vi "Func-엑셀 데이터를 그래프로 출력.vi"() -> ()   [LabVIEW 2015] (continued)
930.01\n930.03\n930.04\n930.06\n930.08\n930.09\n930.11\n930.13\n930.14\n930.16\n930.18\n930.2\n930.21\n930.23\n930.25\n930.26\n930.28\n930.29\n930.31\n930.33\n930.34\n930.36\n930.38\n930.39\n930.41\n930.43\n930.44\n930.46\n930.48\n930.49\n930.51\n930.53\n930.54\n930.56\n930.58\n930.59\n930.61\n930.63\n930.64\n930.66\n930.68\n930.69\n930.71\n930.73\n930.74\n930.76\n930.78\n930.79\n930.81\n930.83\n930.84\n930.86\n930.88\n930.89\n930.91\n930.93\n930.94\n930.96\n930.98\n930.99\n931.01\n931.03\n931.04\n931.06\n931.08\n931.09\n931.11\n931.13\n931.14\n931.16\n931.18\n931.19\n931.21\n931.23\n931.24\n931.26\n931.28\n931.29\n931.31\n931.33\n931.34\n931.36\n931.38\n931.39\n931.41\n931.43\n931.44\n931.46\n931.48\n931.49\n931.51\n931.53\n931.54\n931.56\n931.58\n931.59\n931.61\n931.63\n931.65\n931.66\n931.68\n931.69\n931.71\n931.73\n931.75\n931.76\n931.78\n931.79\n931.81\n931.83\n931.84\n931.86\n931.88\n931.9\n931.91\n931.93\n931.94\n931.96\n931.98\n932\n932.01\n932.03\n932.04\n932.06\n932.08\n932.1\n932.11\n932.13\n932.14\n932.16\n932.18\n932.19\n932.21\n932.23\n932.25\n932.26\n932.28\n932.29\n932.31\n932.33\n932.35\n932.36\n932.38\n932.39\n932.41\n932.43\n932.44\n932.46\n932.48\n932.49\n932.51\n932.53\n932.54\n932.56\n932.58\n932.59\n932.61\n932.63\n932.64\n932.66\n932.68\n932.69\n932.71\n932.73\n932.74\n932.76\n932.78\n932.79\n932.81\n932.83\n932.84\n932.86\n932.88\n932.89\n932.91\n932.93\n932.94\n932.96\n932.98\n932.99\n933.01\n933.03\n933.04\n933.06\n933.08\n933.09\n933.11\n933.13\n933.14\n933.16\n933.18\n933.19\n933.21\n933.23\n933.24\n933.26\n933.28\n933.29\n933.31\n933.33\n933.34\n933.36\n933.38\n933.39\n933.41\n933.43\n933.44\n933.46\n933.48\n933.49\n933.51\n933.53\n933.54\n933.56\n933.58\n933.59\n933.61\n933.63\n933.64\n933.66\n933.68\n933.69\n933.71\n933.73\n933.74\n933.76\n933.78\n933.79\n933.81\n933.83\n933.84\n933.86\n933.88\n933.89\n933.91\n933.93\n933.94\n933.96\n933.98\n933.99\n934.01\n934.03\n934.04\n934.06\n934.08\n934.09\n934.11\n934.13\n934.14\n934.16\n934.18\n934.19\n934.21\n934.23\n934.24\n934.26\n934.28\n934.29\n934.31\n934.33\n934.34\n934.36\n934.38\n934.4\n934.41\n934.43\n934.44\n934.46\n934.48\n934.49\n934.51\n934.53\n934.54\n934.56\n934.58\n934.59\n934.61\n934.63\n934.65\n934.66\n934.68\n934.69\n934.71\n934.73\n934.75\n934.76\n934.78\n934.79\n934.81\n934.83\n934.84\n934.86\n934.88\n934.89\n934.91\n934.93\n934.94\n934.96\n934.98\n935\n935.01\n935.03\n935.04\n935.06\n935.08\n935.1\n935.11\n935.13\n935.14\n935.16\n935.18\n935.2\n935.21\n935.23\n935.24\n935.26\n935.28\n935.29\n935.31\n935.33\n935.35\n935.36\n935.38\n935.39\n935.41\n935.43\n935.45\n935.46\n935.48\n935.49\n935.51\n935.53\n935.54\n935.56\n935.58\n935.6\n935.61\n935.63\n935.64\n935.66\n935.68\n935.7\n935.71\n935.73\n935.74\n935.76\n935.78\n935.8\n935.81\n935.83\n935.84\n935.86\n935.88\n935.89\n935.91\n935.93\n935.94\n935.96\n935.98\n935.99\n936.01\n936.03\n936.04\n936.06\n936.08\n936.09\n936.11\n936.13\n936.14\n936.16\n936.18\n936.19\n936.21\n936.23\n936.24\n936.26\n936.28\n936.29\n936.31\n936.33\n936.34\n936.36\n936.38\n936.39\n936.41\n936.43\n936.44\n936.46\n936.48\n936.49\n936.51\n936.53\n936.54\n936.56\n936.58\n936.59\n936.61\n936.63\n936.64\n936.66\n936.68\n936.69\n936.71\n936.73\n936.74\n936.76\n936.78\n936.79\n936.81\n936.83\n936.84\n936.86\n936.88\n936.89\n936.91\n936.93\n936.94\n936.96\n936.98\n936.99\n937.01\n937.03\n937.04\n937.06\n937.08\n937.09\n937.11\n937.13\n937.14\n937.16\n937.18\n937.19\n937.21\n937.23\n937.24\n937.26\n937.28\n937.29\n937.31\n937.33\n937.34\n937.36\n937.38\n937.4\n937.41\n937.43\n937.44\n937.46\n937.48\n937.5\n937.51\n937.53\n937.54\n937.56\n937.58\n937.59\n937.61\n937.63\n937.65\n937.66\n937.68\n937.69\n937.71\n937.73\n937.75\n937.76\n937.78\n937.79\n937.81\n937.83\n937.85\n937.86\n937.88\n937.89\n937.91\n937.93\n937.94\n937.96\n937.98\n937.99\n938.01\n938.03\n938.04\n938.06\n938.08\n938.1\n938.11\n938.13\n938.14\n938.16\n938.18\n938.2\n938.21\n938.23\n938.24\n938.26\n938.28\n938.29\n938.31\n938.33\n938.35\n938.36\n938.38\n938.39\n938.41\n938.43\n938.45\n938.46\n938.48\n938.49\n938.51\n938.53\n938.55\n938.56\n938.58\n938.59\n938.61\n938.63\n938.64\n938.66\n938.68\n938.7\n938.71\n938.73\n938.74\n938.76\n938.78\n938.8\n938.81\n938.83\n938.84\n938.86\n938.88\n938.89\n938.91\n938.93\n938.95\n938.96\n938.98\n939\n939.01\n939.03\n939.05\n939.06\n939.08\n939.09\n939.11\n939.13\n939.14\n939.16\n939.18\n939.19\n939.21\n939.23\n939.24\n939.26\n939.28\n939.29\n939.31\n939.33\n939.34\n939.36\n939.38\n939.39\n939.41\n939.43\n939.44\n939.46\n939.48\n939.49\n939.51\n939.53\n939.54\n939.56\n939.58\n939.59\n939.61\n939.63\n939.64\n939.66\n939.68\n939.69\n939.71\n939.73\n939.74\n939.76\n939.78\n939.79\n939.81\n939.83\n939.84\n939.86\n939.88\n939.89\n939.91\n939.93\n939.94\n939.96\n939.98\n939.99\n940.01\n940.03\n940.04\n940.06\n940.08\n940.09\n940.11\n940.13\n940.14\n940.16\n940.18\n940.19\n940.21\n940.23\n940.24\n940.26\n940.28\n940.29\n940.31\n940.33\n940.34\n940.36\n940.38\n940.39\n940.41\n940.43\n940.44\n940.46\n940.48\n940.5\n940.51\n940.53\n940.54\n940.56\n940.58\n940.59\n940.61\n940.63\n940.64\n940.66\n940.68\n940.69\n940.71\n940.73\n940.75\n940.76\n940.78\n940.79\n940.81\n940.83\n940.85\n940.86\n940.88\n940.89\n940.91\n940.93\n940.94\n940.96\n940.98\n940.99\n941.01\n941.03\n941.04\n941.06\n941.08\n941.1\n941.11\n941.13\n941.14\n941.16\n941.18\n941.2\n941.21\n941.23\n941.24\n941.26\n941.28\n941.29\n941.31\n941.33\n941.34\n941.36\n941.38\n941.39\n941.41\n941.43\n941.45\n941.46\n941.48\n941.49\n941.51\n941.53\n941.54\n941.56\n941.58\n941.59\n941.61\n941.63\n941.64\n941.66\n941.68\n941.69\n941.71\n941.73\n941.74\n941.76\n941.78\n941.79\n941.81\n941.83\n941.84\n941.86\n941.88\n941.89\n941.91\n941.93\n941.94\n941.96\n941.98\n942\n942.01\n942.03\n942.04\n942.06\n942.08\n942.09\n942.11\n942.13\n942.14\n942.16\n942.18\n942.19\n942.21\n942.23\n942.24\n942.26\n942.28\n942.29\n942.31\n942.33\n942.34\n942.36\n942.38\n942.39\n942.41\n942.43\n942.44\n942.46\n942.48\n942.49\n942.51\n942.53\n942.54\n942.56\n942.58\n942.59\n942.61\n942.63\n942.64\n942.66\n942.68\n942.69\n942.71\n942.73\n942.74\n942.76\n942.78\n942.79\n942.81\n942.83\n942.84\n942.86\n942.88\n942.89\n942.91\n942.93\n942.94\n942.96\n942.98\n942.99\n943.01\n943.03\n943.04\n943.06\n943.08\n943.09\n943.11\n943.13\n943.14\n943.16\n943.18\n943.19\n943.21\n943.23\n943.24\n943.26\n943.28\n943.29\n943.31\n943.33\n943.34\n943.36\n943.38\n943.39\n943.41\n943.43\n943.44\n943.46\n943.48\n943.5\n943.51\n943.53\n943.54\n943.56\n943.58\n943.59\n943.61\n943.63\n943.64\n943.66\n943.68\n943.69\n943.71\n943.73\n943.74\n943.76\n943.78\n943.79\n943.81\n943.83\n943.85\n943.86\n943.88\n943.89\n943.91\n943.93\n943.95\n943.96\n943.98\n943.99\n944.01\n944.03\n944.04\n944.06\n944.08\n944.1\n944.11\n944.13\n944.14\n944.16\n944.18\n944.2\n944.21\n944.23\n944.24\n944.26\n944.28\n944.29\n944.31\n944.33\n944.34\n944.36\n944.38\n944.39\n944.41\n944.43\n944.44\n944.46\n944.48\n944.49\n944.51\n944.53\n944.55\n944.56\n944.58\n944.59\n944.61\n944.63\n944.64\n944.66\n944.68\n944.69\n944.71\n944.73\n944.74\n944.76\n944.78\n944.79\n944.81\n944.83\n944.84\n944.86\n944.88\n944.89\n944.91\n944.93\n944.94\n944.96\n944.98\n944.99\n945.01\n945.03\n945.04\n945.06\n945.08\n945.09\n945.11\n945.13\n945.14\n945.16\n945.18\n945.19\n945.21\n945.23\n945.24\n945.26\n945.28\n945.29\n945.31\n945.33\n945.34\n945.36\n945.38\n945.39\n945.41\n945.43\n945.44\n945.46\n945.48\n945.49\n945.51\n945.53\n945.54\n945.56\n945.58\n945.59\n945.61\n945.63\n945.64\n945.66\n945.68\n945.69\n945.71\n945.73\n945.74\n945.76\n945.78\n945.79\n945.81\n945.83\n945.84\n945.86\n945.88\n945.89\n945.91\n945.93\n945.94\n945.96\n945.98\n945.99\n946.01\n946.03\n946.04\n946.06\n946.08\n946.09\n946.11\n946.13\n946.14\n946.16\n946.18\n946.19\n946.21\n946.23\n946.25\n946.26\n946.28\n946.29\n946.31\n946.33\n946.34\n946.36\n946.38\n946.39\n946.41\n946.43\n946.44\n946.46\n946.48\n946.49\n946.51\n946.53\n946.54\n946.56\n946.58\n946.6\n946.61\n946.63\n946.64\n946.66\n946.68\n946.69\n946.71\n946.73\n946.74\n946.76\n946.78\n946.79\n946.81\n946.83\n946.85\n946.86\n946.88\n946.89\n946.91\n946.93\n946.95\n946.96\n946.98\n946.99\n947.01\n947.03\n947.04\n947.06\n947.08\n947.09\n947.11\n947.13\n947.14\n947.16\n947.18\n947.2\n947.21\n947.23\n947.24\n947.26\n947.28\n947.3\n947.31\n947.33\n947.34\n947.36\n947.38\n947.39\n947.41\n947.43\n947.44\n947.46\n947.48\n947.49\n947.51\n947.53\n947.55\n947.56\n947.58\n947.59\n947.61\n947.63\n947.65\n947.66\n947.68\n947.69\n947.71\n947.73\n947.74\n947.76\n947.78\n947.79\n947.81\n947.83\n947.84\n947.86\n947.88\n947.89\n947.91\n947.93\n947.94\n947.96\n947.98\n947.99\n948.01\n948.03\n948.04\n948.06\n948.08\n948.09\n948.11\n948.13\n948.14\n948.16\n948.18\n948.19\n948.21\n948.23\n948.24\n948.26\n948.28\n948.29\n948.31\n948.33\n948.35\n948.36\n948.38\n948.39\n948.41\n948.43\n948.44\n948.46\n948.48\n948.49\n948.51\n948.53\n948.54\n948.56\n948.58\n948.59\n948.61\n948.63\n948.64\n948.66\n948.68\n948.69\n948.71\n948.73\n948.74\n948.76\n948.78\n948.79\n948.81\n948.83\n948.84\n948.86\n948.88\n948.89\n948.91\n948.93\n948.94\n948.96\n948.98\n949\n949.01\n949.03\n949.04\n949.06\n949.08\n949.09\n949.11\n949.13\n949.14\n949.16\n949.18\n949.19\n949.21\n949.23\n949.25\n949.26\n949.28\n949.29\n949.31\n949.33\n949.34\n949.36\n949.38\n949.39\n949.41\n949.43\n949.44\n949.46\n949.48\n949.49\n949.51\n949.53\n949.54\n949.56\n949.58\n949.6\n949.61\n949.63\n949.64\n949.66\n949.68\n949.7\n949.71\n949.73\n949.74\n949.76\n949.78\n949.79\n949.81\n949.83\n949.85\n949.86\n949.88\n949.89\n949.91\n949.93\n949.95\n949.96\n949.98\n949.99\n950.01\n950.03\n950.04\n950.06\n950.08\n950.09\n950.11\n950.13\n950.14\n950.16\n950.18\n950.2\n950.21\n950.23\n950.24\n950.26\n950.28\n950.3\n950.31\n950.33\n950.34\n950.36\n950.38\n950.39\n950.41\n950.43\n950.44\n950.46\n950.48\n950.49\n950.51\n950.53\n950.55\n950.56\n950.58\n950.59\n950.61\n950.63\n950.65\n950.66\n950.68\n950.69\n950.71\n950.73\n950.75\n950.76\n950.78\n950.79\n950.81\n950.83\n950.84\n950.86\n950.88\n950.89\n950.91\n950.93\n950.94\n950.96\n950.98\n951\n951.01\n951.03\n951.04\n951.06\n951.08\n951.1\n951.11\n951.13\n951.15\n951.16\n951.18\n951.19\n951.21\n951.23\n951.24\n951.26\n951.28\n951.29\n951.31\n951.33\n951.34\n951.36\n951.38\n951.39\n951.41\n951.43\n951.44\n951.46\n951.48\n951.49\n951.51\n951.53\n951.54\n951.56\n951.58\n951.59\n951.61\n951.63\n951.64\n951.66\n951.68\n951.69\n951.71\n951.73\n951.74\n951.76\n951.78\n951.79\n951.81\n951.83\n951.84\n951.86\n951.88\n951.89\n951.91\n951.93\n951.94\n951.96\n951.98\n951.99\n952.01\n952.03\n952.04\n952.06\n952.08\n952.09\n952.11\n952.13\n952.14\n952.16\n952.18\n952.19\n952.21\n952.23\n952.24\n952.26\n952.28\n952.29\n952.31\n952.33\n952.35\n952.36\n952.38\n952.39\n952.41\n952.43\n952.44\n952.46\n952.48\n952.49\n952.51\n952.53\n952.54\n952.56\n952.58\n952.59\n952.61\n952.63\n952.64\n952.66\n952.68\n952.7\n952.71\n952.73\n952.74\n952.76\n952.78\n952.79\n952.81\n952.83\n952.84\n952.86\n952.88\n952.89\n952.91\n952.93\n952.95\n952.96\n952.98\n952.99\n953.01\n953.03\n953.05\n953.06\n953.08\n953.09\n953.11\n953.13\n953.14\n953.16\n953.18\n953.19\n953.21\n953.23\n953.24\n953.26\n953.28\n953.3\n953.31\n953.33\n953.34\n953.36\n953.38\n953.4\n953.41\n953.43\n953.44\n953.46\n953.48\n953.49\n953.51\n953.53\n953.54\n953.56\n953.58\n953.59\n953.61\n953.63\n953.64\n953.66\n953.68\n953.69\n953.71\n953.73\n953.74\n953.76\n953.78\n953.79\n953.81\n953.83\n953.84\n953.86\n953.88\n953.89\n953.91\n953.93\n953.94\n953.96\n953.98\n953.99\n954.01\n954.03\n954.04\n954.06\n954.08\n954.09\n954.11\n954.13\n954.14\n954.16\n954.18\n954.2\n954.21\n954.23\n954.24\n954.26\n954.28\n954.29\n954.31\n954.33\n954.34\n954.36\n954.38\n954.39\n954.41\n954.43\n954.44\n954.46\n954.48\n954.49\n954.51\n954.53\n954.54\n954.56\n954.58\n954.59\n954.61\n954.63\n954.64\n954.66\n954.68\n954.69\n954.71\n954.73\n954.74\n954.76\n954.78\n954.79\n954.81\n954.83\n954.84\n954.86\n954.88\n954.89\n954.91\n954.93\n954.94\n954.96\n954.98\n954.99\n955.01\n955.03\n955.04\n955.06\n955.08\n955.1\n955.11\n955.13\n955.14\n955.16\n955.18\n955.19\n955.21\n955.23\n955.24\n955.26\n955.28\n955.29\n955.31\n955.33\n955.34\n955.36\n955.38\n955.39\n955.41\n955.43\n955.45\n955.46\n955.48\n955.49\n955.51\n955.53\n955.54\n955.56\n955.58\n955.59\n955.61\n955.63\n955.64\n955.66\n955.68\n955.69\n955.71\n955.73\n955.74\n955.76\n955.78\n955.8\n955.81\n955.83\n955.84\n955.86\n955.88\n955.89\n955.91\n955.93\n955.94\n955.96\n955.98\n955.99\n956.01\n956.03\n956.05\n956.06\n956.08\n956.09\n956.11\n956.13\n956.15\n956.16\n956.18\n956.19\n956.21\n956.23\n956.25\n956.26\n956.28\n956.3\n956.31\n956.33\n956.34\n956.36\n956.38\n956.39\n956.41\n956.43\n956.44\n956.46\n956.48\n956.5\n956.51\n956.53\n956.54\n956.56\n956.58\n956.6\n956.61\n956.63\n956.64\n956.66\n956.68\n956.69\n956.71\n956.73\n956.75\n956.76\n956.78\n956.79\n956.81\n956.83\n956.85\n956.86\n956.88\n956.89\n956.91\n956.93\n956.94\n956.96\n956.98\n956.99\n957.01\n957.03\n957.04\n957.06\n957.08\n957.09\n957.11\n957.13\n957.14\n957.16\n957.18\n957.2\n957.21\n957.23\n957.24\n957.26\n957.28\n957.29\n957.31\n957.33\n957.34\n957.36\n957.38\n957.39\n957.41\n957.43\n957.45\n957.46\n957.48\n957.49\n957.51\n957.53\n957.54\n957.56\n957.58\n957.59\n957.61\n957.63\n957.64\n957.66\n957.68\n957.69\n957.71\n957.73\n957.74\n957.76\n957.78\n957.79\n957.81\n957.83\n957.84\n957.86\n957.88\n957.89\n957.91\n957.93\n957.94\n957.96\n957.98\n957.99\n958.01\n958.03\n958.04\n958.06\n958.08\n958.09\n958.11\n958.13\n958.14\n958.16\n958.18\n958.19\n958.21\n958.23\n958.24\n958.26\n958.28\n958.29\n958.31\n958.33\n958.34\n958.36\n958.38\n958.39\n958.41\n958.43\n958.44\n958.46\n958.48\n958.49\n958.51\n958.53\n958.54\n958.56\n958.58\n958.59\n958.61\n958.63\n958.64\n958.66\n958.68\n958.69\n958.71\n958.73\n958.74\n958.76\n958.78\n958.8\n958.81\n958.83\n958.84\n958.86\n958.88\n958.9\n958.91\n958.93\n958.94\n958.96\n958.98\n958.99\n959.01\n959.03\n959.04\n959.06\n959.08\n959.09\n959.11\n959.13\n959.15\n959.16\n959.18\n959.19\n959.21\n959.23\n959.25\n959.26\n959.28\n959.29\n959.31\n959.33\n959.34\n959.36\n959.38\n959.39\n959.41\n959.43\n959.44\n959.46\n959.48\n959.49\n959.51\n959.53\n959.54\n959.56\n959.58\n959.6\n959.61\n959.63\n959.64\n959.66\n959.68\n959.69\n959.71\n959.73\n959.74\n959.76\n959.78\n959.79\n959.81\n959.83\n959.84\n959.86\n959.88\n959.89\n959.91\n959.93\n959.94\n959.96\n959.98\n959.99\n960.01\n960.03\n960.04\n960.06\n960.08\n960.1\n960.11\n960.13\n960.14\n960.16\n960.18\n960.2\n960.21\n960.23\n960.24\n960.26\n960.28\n960.29\n960.31\n960.33\n960.34\n960.36\n960.38\n960.39\n960.41\n960.43\n960.44\n960.46\n960.48\n960.49\n960.51\n960.53\n960.54\n960.56\n960.58\n960.59\n960.61\n960.63\n960.64\n960.66\n960.68\n960.69\n960.71\n960.73\n960.74\n960.76\n960.78\n960.79\n960.81\n960.83\n960.84\n960.86\n960.88\n960.89\n960.91\n960.93\n960.94\n960.96\n960.98\n960.99\n961.01\n961.03\n961.04\n961.06\n961.08\n961.09\n961.11\n961.13\n961.14\n961.16\n961.18\n961.2\n961.21\n961.23\n961.24\n961.26\n961.28\n961.29\n961.31\n961.33\n961.34\n961.36\n961.38\n961.39\n961.41\n961.43\n961.44\n961.46\n961.48\n961.49\n961.51\n961.53\n961.55\n961.56\n961.58\n961.59\n961.61\n961.63\n961.64\n961.66\n961.68\n961.69\n961.71\n961.73\n961.74\n961.76\n961.78\n961.79\n961.81\n961.83\n961.84\n961.86\n961.88\n961.9\n961.91\n961.93\n961.94\n961.96\n961.98\n961.99\n962.01\n962.03\n962.04\n962.06\n962.08\n962.09\n962.11\n962.13\n962.15\n962.16\n962.18\n962.19\n962.21\n962.23\n962.25\n962.26\n962.28\n962.29\n962.31\n962.33\n962.35\n962.36\n962.38\n962.39\n962.41\n962.43\n962.44\n962.46\n962.48\n962.5\n962.51\n962.53\n962.54\n962.56\n962.58\n962.6\n962.61\n962.63\n962.64\n962.66\n962.68\n962.69\n962.71\n962.73\n962.74\n962.76\n962.78\n962.79\n962.81\n962.83\n962.84\n962.86\n962.88\n962.89\n962.91\n962.93\n962.95\n962.96\n962.98\n962.99\n963.01\n963.03\n963.04\n963.06\n963.08\n963.1\n963.11\n963.13\n963.14\n963.16\n963.18\n963.19\n963.21\n963.23\n963.24\n963.26\n963.28\n963.3\n963.31\n963.33\n963.34\n963.36\n963.38\n980.53\n980.71\n980.87\n981.04\n981.21\n981.37\n981.54\n981.71\n981.88\n982.05\n982.21\n982.38\n982.55\n982.72\n982.88\n983.05\n983.21\n983.39\n983.56\n983.72\n983.89\n984.06\n984.22\n984.39\n984.56\n984.72\n984.89\n985.06\n985.22\n985.4\n985.56\n985.73\n985.9\n986.06\n986.23\n986.4\n986.56\n986.73\n986.91\n987.07\n987.24\n987.41\n987.57\n987.74\n987.91\n988.07\n988.24\n988.41\n988.57\n988.74\n988.91\n989.07\n989.24\n989.41\n989.57\n989.74\n989.91\n990.07\n990.24\n990.41\n990.57\n990.74\n990.91\n991.07\n991.24\n991.41\n991.57\n991.74\n991.91\n992.07\n992.25\n992.41\n992.58\n992.75\n992.91\n993.08\n993.25\n993.41\n993.58\n993.75\n993.91\n994.08\n994.25\n994.41\n994.58\n994.75\n994.91\n995.08\n995.25\n995.41\n995.58\n995.75\n995.91\n996.08\n996.25\n996.41\n996.58\n996.75\n996.91\n997.08\n997.25\n997.41\n997.58\n997.75\n997.91\n998.08\n998.25\n998.42\n998.59\n998.76\n998.92\n999.09\n999.26\n999.42\n999.59\n999.76\n999.92\n1000.09\n1000.26\n1000.42\n1000.59\n1000.76\n1000.92\n1001.09\n1001.26\n1001.42\n1001.59\n1001.76\n1001.92\n1002.09\n1002.26\n1002.42\n1002.59\n1002.76\n1002.92\n1003.09\n1003.26\n1003.42\n1003.59\n1003.76\n1003.92\n1004.09\n1004.26\n1004.43\n1004.6\n1004.76\n1004.93\n1005.1\n1005.26\n1005.43\n1005.61\n1005.77\n1005.95\n1006.11\n1006.28\n1006.45\n1006.61\n1006.78\n1006.95\n1007.11\n1007.28\n1007.45\n1007.61\n1007.78\n1007.95\n1008.11\n1008.28\n1008.45\n1008.62\n1008.78\n1008.95\n1009.11\n1009.28\n1009.45\n1009.62\n1009.79\n1009.96\n1010.12\n1010.29\n1010.46\n1010.62\n1010.79\n1010.96\n1011.12\n1011.29\n1011.46\n1011.62\n1011.79\n1011.96\n1012.12\n1012.29\n1012.46\n1012.62\n1012.79\n1012.96\n1013.12\n1013.29\n1013.46\n1013.62\n1013.79\n1013.96\n1014.13\n1014.3\n1014.46\n1014.63\n1014.8\n1014.96\n1015.13\n1015.3\n1015.46\n1015.63\n1015.8\n1015.96\n1016.14\n1016.31\n1016.47\n1016.64\n1016.81\n1016.97\n1017.14\n1017.31\n1017.47\n1017.64\n1017.81\n1017.97\n1018.14\n1018.31\n1018.47\n1018.64\n1018.81\n1018.97\n1019.14\n1019.31\n1019.47\n1019.64\n1019.81\n1019.97\n1020.14\n1020.31\n1020.47\n1020.64\n1020.81\n1020.97\n1021.14\n1021.31\n1021.47\n1021.64\n1021.81\n1021.97\n1022.14\n1022.31\n1022.48\n1022.65\n1022.81\n1022.98\n1023.15\n1023.32\n1023.48\n1023.65\n1023.81\n1023.98\n1024.14\n1024.14\n1024.16\n1024.18\n1024.19\n1024.21\n1024.23\n1024.24\n1024.26\n1024.28\n1024.29\n1024.31\n1024.33\n1024.34\n1024.36\n1024.38\n1024.39\n1024.41\n1024.43\n1024.44\n1024.46\n1024.48\n1024.49\n1024.51\n1024.53\n1024.54\n1024.56\n1024.58\n1024.59\n1024.61\n1024.63\n1024.64\n1024.66\n1024.68\n1024.69\n1024.71\n1024.73\n1024.74\n1024.76\n1024.78\n1024.79\n1024.81\n1024.83\n1024.84\n1024.86\n1024.88\n1024.89\n1024.91\n1024.93\n1024.94\n1024.96\n1024.98\n1024.99\n1025.01\n1025.03\n1025.04\n1025.06\n1025.08\n1025.09\n1025.11\n1025.13\n1025.14\n1025.16\n1025.18\n1025.19\n1025.21\n1025.23\n1025.24\n1025.26\n1025.28\n1025.29\n1025.31\n1025.33\n1025.35\n1025.36\n1025.38\n1025.39\n1025.41\n1025.43\n1025.44\n1025.46\n1025.48\n1025.49\n1025.51\n1025.53\n1025.54\n1025.56\n1025.58\n1025.6\n1025.61\n1025.63\n1025.64\n1025.66\n1025.68\n1025.7\n1025.71\n1025.73\n1025.74\n1025.76\n1025.78\n1025.79\n1025.81\n1025.83\n1025.84\n1025.86\n1025.88\n1025.89\n1025.91\n1025.93\n1025.95\n1025.96\n1025.98\n1025.99\n1026.01\n1026.03\n1026.05\n1026.06\n1026.08\n1026.09\n1026.11\n1026.13\n1026.15\n1026.16\n1026.18\n1026.19\n1026.21\n1026.23\n1026.24\n1026.26\n1026.28\n1026.29\n1026.31\n1026.33\n1026.34\n1026.36\n1026.38\n1026.39\n1026.41\n1026.43\n1026.44\n1026.46\n1026.48\n1026.49\n1026.51\n1026.53\n1026.54\n1026.56\n1026.58\n1026.59\n1026.61\n1026.63\n1026.64\n1026.66\n1026.68\n1026.69\n1026.71\n1026.73\n1026.74\n1026.76\n1026.78\n1026.79\n1026.81\n1026.83\n1026.84\n1026.86\n1026.88\n1026.89\n1026.91\n1026.93\n1026.94\n1026.96\n1026.98\n1026.99\n1027.01\n1027.03\n1027.04\n1027.06\n1027.08\n1027.09\n1027.11\n1027.13\n1027.14\n1027.16\n1027.18\n1027.19\n1027.21\n1027.23\n1027.24\n1027.26\n1027.28\n1027.29\n1027.31\n1027.33\n1027.34\n1027.36\n1027.38\n1027.39\n1027.41\n1027.43\n1027.44\n1027.46\n1027.48\n1027.49\n
